vi "Graphing Engine.vi"   [LabVIEW 2013]
types:
  T1 = cluster{"Graph Height1":dbl, "Graph Height2":dbl, "Graph Time":dbl}
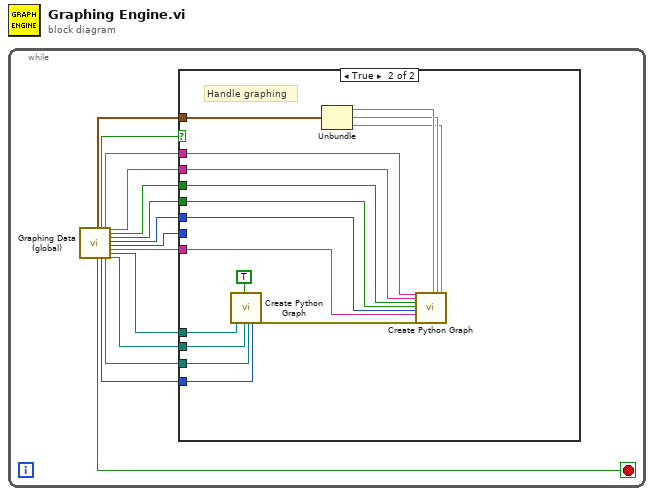
[diagram p0: block diagram]
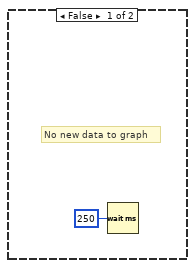
[diagram p2: hidden frame]
diagram:
  n1 = while {
    stop <- w2 stop-if-true
    n2 = call "Graphing Data (global).vi"() -> ("Graph Settings OUT"=w1:T1, "STOP"=w2:bool, "Data Ready?"=w14:bool, "Data Start Index"=w10:u32, "File Name"=w13:string, "Python Script Directory"=w9:path, "Title"=w12:string, "Main Side"=w11:bool, "Wet Test"=w3:bool, "Y-Axis Max"=w4:i32, "Data End Index"=w5:i32, "LS Series"=w6:string, "Data Base Path"=w7:path, "Tolerances Path"=w8:path)  [unwired: 14 in]
    n3 = case shown="True" w14 {
      tunnel: w10 -> [_ w30]
      tunnel: w7 -> [_ w29]
      tunnel: w8 -> [_ w28]
      tunnel: w9 -> [_ w27]
      tunnel: w13 -> [_ w25]
      tunnel: w12 -> [_ w24]
      tunnel: w11 -> [_ w23]
      tunnel: w3 -> [_ w22]
      tunnel: w4 -> [_ w21]
      tunnel: w5 -> [_ _]
      tunnel: w6 -> [_ w16]
      tunnel: w1 -> [_ w20]
      frame False {
        # "No new data to graph"
        n4 = Wait (ms)(milliseconds to wait=u32 250) -> ()  [unwired: 1 out]
      }
      frame True {
        # "Handle graphing"
        n5 = call "Create Python Graph.vi"("Data Base Path"=w29, "Init (F)"=TRUE, "Tolerances Path"=w28, "Python Script Directory"=w27, "Data Start Index"=w30) -> ("Error OUT"=w26:errorcluster)  [unwired: 21 in, 1 out]
        n6 = Unbundle(w20) -> ("Graph Height1"=w19:dbl, "Graph Height2"=w18:dbl, "Graph Time"=w17:dbl)
        n7 = call "Create Python Graph.vi"("File Name"=w25, "Title"=w24, "Main Side"=w23, "Wet Test"=w22, "Y-Axis Max"=w21, "LS Series"=w16, "Error IN"=w26, "X-Axis Min"=w19, "X-Axis Max (Height)"=w18, "X-Axis Max (Time)"=w17) -> ()  [unwired: 16 in, 2 out]
      }
    }
  }
